vi "Sand Fall Till the Source.vi"(3 "Possible Movements":cdb[](array[numeric]), 4 "Sand Source Coordinates":cdb, 5 "Rock Grid":set{cdb}(c389)) -> (0 "Bounds":T1, 1 "Sand Fall steps":T2(array[cluster]), 2 "Sand Grid":set{cdb}(c389))   [LabVIEW 2020, in "AoC 2022.lvlib"]
uses:
  AoC 2022.lvlib
panel:
  out "size":i32
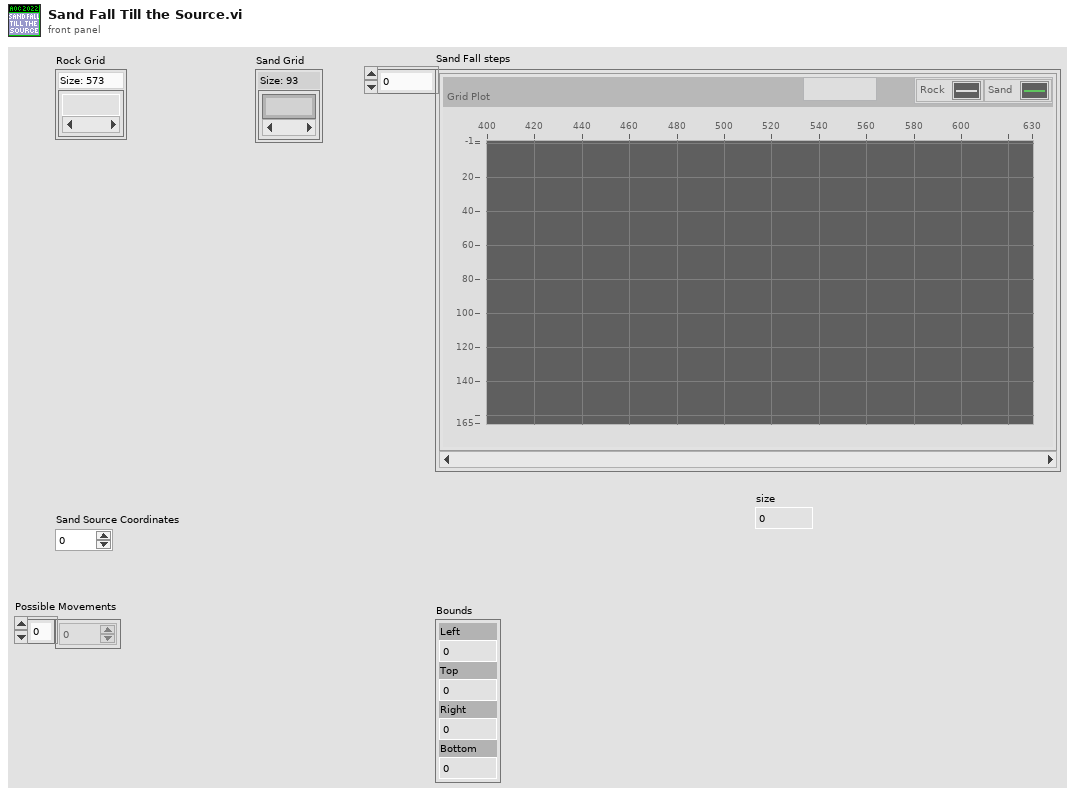
[diagram p1: front panel]
types:
  T1 = cluster{"Left":i16, "Top":i16, "Right":i16, "Bottom":i16}
  T2 = cluster{"Grid Plot":cluster{cluster{i32, i32}[]}[]}[]
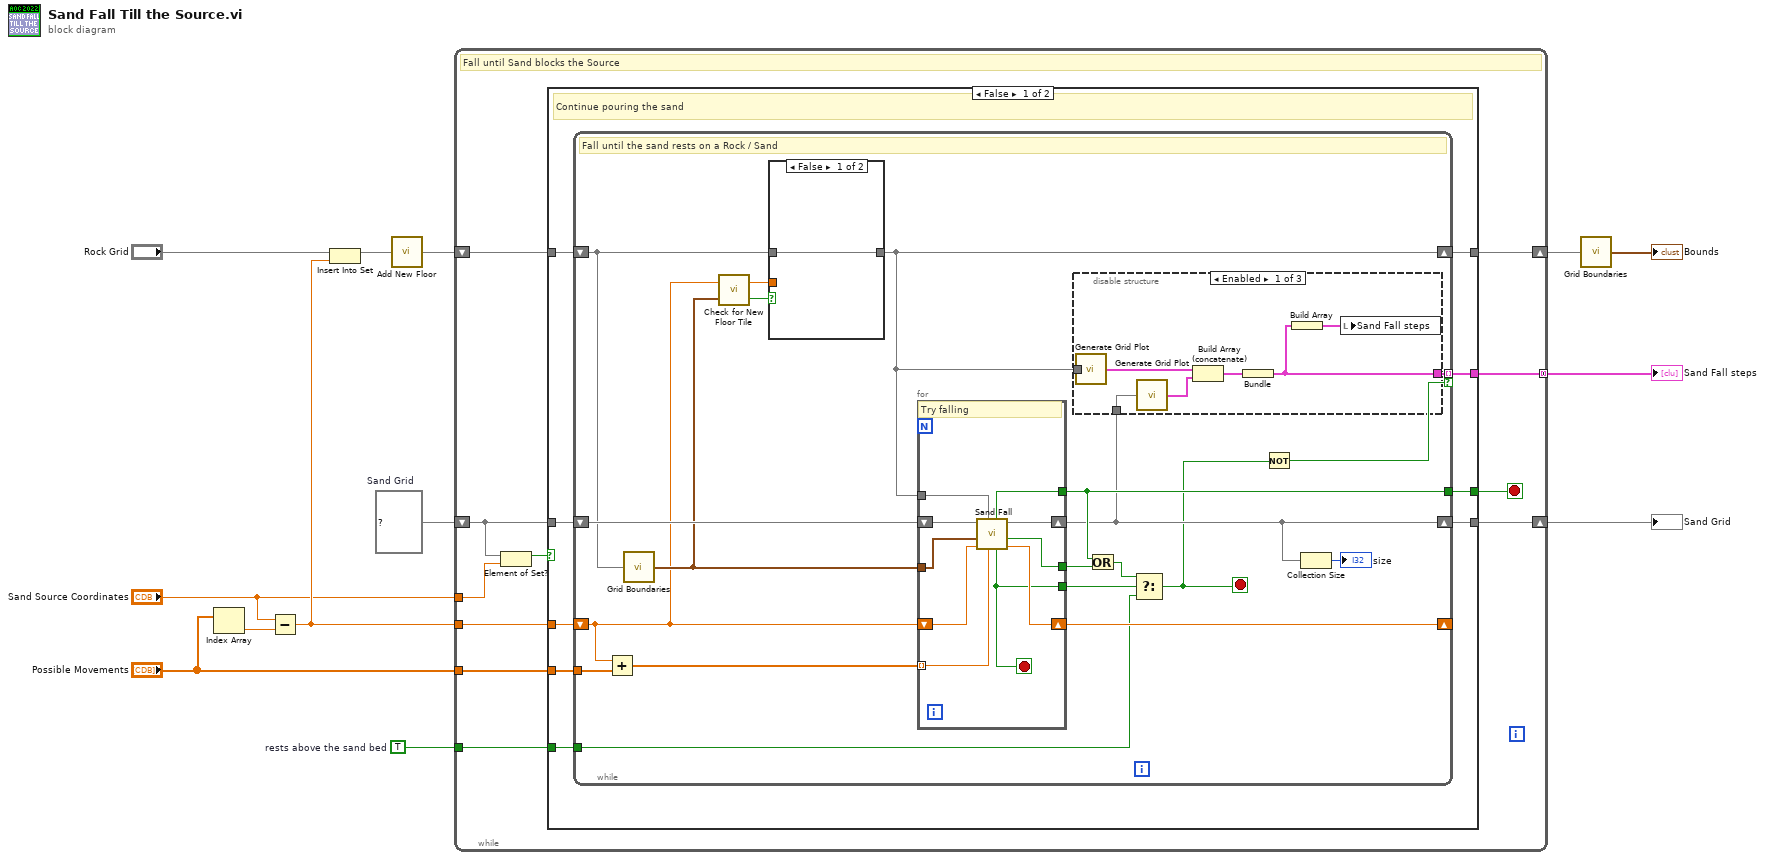
[diagram p0: block diagram]
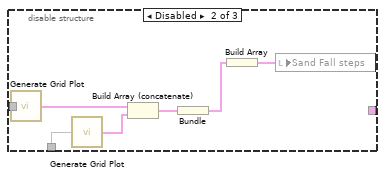
[diagram p2: hidden frame]
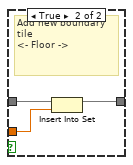
[diagram p4: hidden frame]
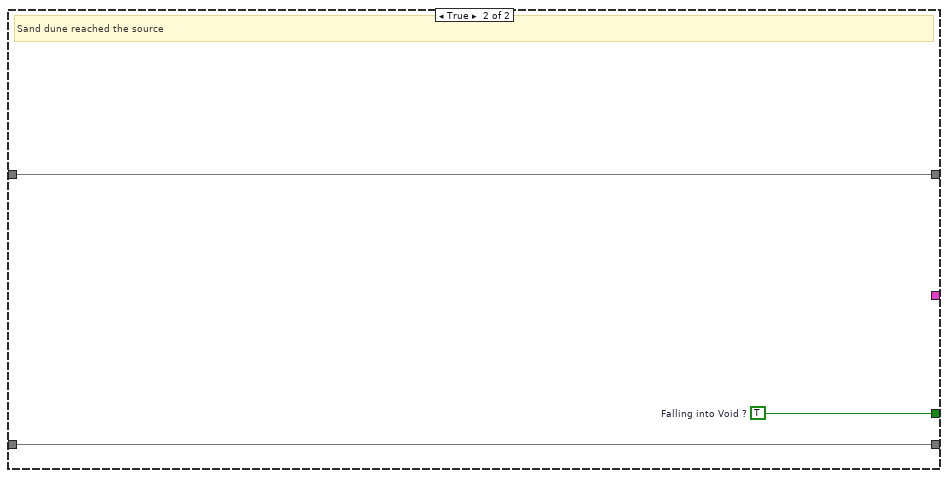
[diagram p5: hidden frame]
diagram:
  w11 = TRUE  # rests above the sand bed
  w12 = set{cdb} {}  # Sand Grid
  n1 = Index Array(array="Possible Movements") -> (element=w4:cdb)  [unwired: 1 in]
  n2 = Subtract(x="Sand Source Coordinates", y=w4) -> (x-y=w2:cdb)
  n3 = Insert Into Set(10:w2, 11:"Rock Grid") -> (3:w9:set{cdb})  [unwired: 1 out]
  n4 = call "Add New Floor.vi"("Rock Grid in"=w9) -> ("Rock Grid out"=w8:set{cdb})
  n5 = while {
    shift-right: [w21] -> w13
    shift-left: w12 -> [w17]
    tunnel: w2 -> [w15]
    tunnel: "Possible Movements" -> [w24]
    tunnel: [w22] -> w3 mode=concatenating
    tunnel: w11 -> [w20]
    shift-right: [w18] -> w7
    shift-left: w8 -> [w19]
    tunnel: "Sand Source Coordinates" -> [w14]
    stop <- w23 stop-if-true
    # "Fall until Sand blocks the Source"
    n6 = Element of Set?(10:w14, 11:w17) -> (3:w16:bool)
    n7 = case shown="False" w16 {
      tunnel: w24 -> [w33 _]
      tunnel: [w32 w83] -> w23
      tunnel: [w31 _] -> w22
      tunnel: [w30 w82] -> w21
      tunnel: w20 -> [w29 _]
      tunnel: w19 -> [w28 w84]
      tunnel: [w27 w84] -> w18
      tunnel: w17 -> [w25 w82]
      tunnel: w15 -> [w26 _]
      frame False {
        # "Continue pouring the sand"
        n8 = while {
          shift-right: [w35] -> w30
          shift-left: w25 -> [w52]
          shift-right: [w53] -> _
          shift-left: w26 -> [w39]
          tunnel: w33 -> [w51]
          tunnel: [w48] -> w32
          tunnel: [w37] -> w31 mode=indexing if=w45
          tunnel: w29 -> [w44]
          shift-right: [w43] -> w27
          shift-left: w28 -> [w42]
          stop <- w34 stop-if-true
          # "Fall until the sand rests on a Rock / Sand"
          n9 = Add(x=w39, y=w51) -> (x+y=w50:cdb[])
          n10 = call "Grid Boundaries.vi"("Grid"=w42) -> ("Bounds"=w41:T1)
          n11 = call "Check for New Floor Tile.vi"("Bounds"=w41, "Current Location"=w39) -> ("Add floor tile ?"=w40:bool, "New Floor Tile"=w38:cdb)
          n12 = case shown="False" w40 {
            tunnel: w42 -> [w68 w71]
            tunnel: [w68 w70] -> w43
            tunnel: w38 -> [_ w69]
            frame False {
            }
            frame True {
              # "Add new boundary tile\n<- Floor ->"
              n13 = Insert Into Set(10:w69, 11:w71) -> (3:w70:set{cdb})  [unwired: 1 out]
            }
          }
          n14 = for {
            tunnel: w43 -> [w79]
            tunnel: w41 -> [w77]
            shift-right: [w78] -> w53
            shift-left: w39 -> [w76]
            shift-right: [w81] -> w35
            shift-left: w52 -> [w80]
            tunnel: w50 -> [w75] mode=indexing
            tunnel: [w74] -> w49
            tunnel: [w72] -> w48
            tunnel: [w73] -> w47
            stop <- w73 stop-if-true
            # "Try falling"
            n15 = call "Sand Fall.vi"("Next Location"=w75, "Rock Grid"=w79, "Current Location in"=w76, "Bounds"=w77, "Sand Grid in"=w80) -> ("Current Location out"=w78:cdb, "Sand Reached Resting Position ?"=w74:bool, "Sand Grid out"=w81:set{cdb}, "Arrived at Decision ?"=w73:bool, "Falling into Void ?"=w72:bool)  [unwired: 2 in]
          }
          n16 = disable-structure shown="Enabled" {
            disable-tunnel: w43 -> [w58 w65 _]
            disable-tunnel: [w56 _ _] -> w37
            disable-tunnel: w35 -> [w54 w61 _]
            frame Enabled {
              n17 = call "Generate Grid Plot.vi"("Grid"=w58) -> ("Grid Plot"=w59:cluster{cluster{i32, i32}[]}[])
              n18 = call "Generate Grid Plot.vi"("Grid"=w54) -> ("Grid Plot"=w60:cluster{cluster{i32, i32}[]}[])
              n19 = Build Array (concatenate)(w59, w60) -> (w57:cluster{cluster{i32, i32}[]}[])
              n20 = Bundle(w57) -> (w56:cluster{cluster{cluster[]}[]})  [unwired: 1 in]
              n21 = Build Array(w56) -> (w55:cluster{cluster{cluster[]}[]}[])
              n22 = local write "Sand Fall steps"(w55) -> ()
            }
            frame Disabled {
              n23 = call "Generate Grid Plot.vi"("Grid"=w65) -> ("Grid Plot"=w66:cluster{cluster{i32, i32}[]}[])
              n24 = call "Generate Grid Plot.vi"("Grid"=w61) -> ("Grid Plot"=w67:cluster{cluster{i32, i32}[]}[])
              n25 = Build Array (concatenate)(w66, w67) -> (w64:cluster{cluster{i32, i32}[]}[])
              n26 = Bundle(w64) -> (w63:cluster{cluster{cluster[]}[]})  [unwired: 1 in]
              n27 = Build Array(w63) -> (w62:cluster{cluster{cluster[]}[]}[])
              n28 = local write "Sand Fall steps"(w62) -> ()
            }
            frame Disabled {
            }
          }
          n29 = Or(x=w48, y=w49) -> (x .or. y?=w46:bool)
          n30 = Select(t=w46, s=w47, f=w44) -> (s? t:f=w34:bool)
          n31 = Not(x=w34) -> (.not. x?=w45:bool)
          n32 = Collection Size(1:w35) -> (0:→"size":i32)
        }
      }
      frame True {
        w83 = TRUE  # Falling into Void ?
        # "Sand dune reached the source"
      }
    }
  }
  "Sand Grid" <- w13
  "Sand Fall steps" <- w3
  n33 = call "Grid Boundaries.vi"("Grid"=w7) -> ("Bounds"=→"Bounds":T1)
